vi "YKMW100 Clear Output Buffer.vi"(0 "VISA session":refnum<visa-resource-name>="MW100", 11 "error in (no error)":errorcluster) -> (4 "dup VISA session":refnum<visa-resource-name>, 15 "error out":errorcluster)   [LabVIEW 2023]
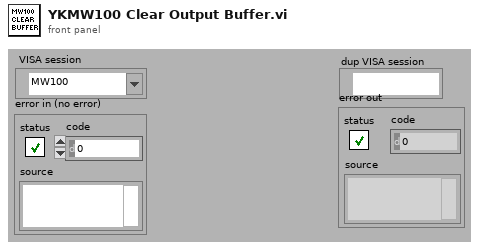
[diagram p1: front panel]
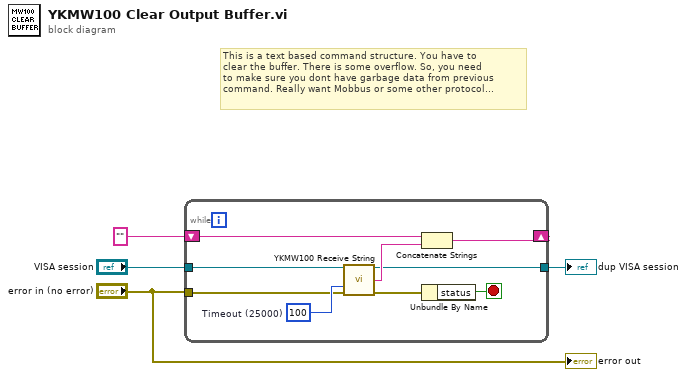
[diagram p0: block diagram]
diagram:
  # "This is a text based command structure. You have to \nclear the buffer. There is some overflow. So, you need\nto make sure you dont have garbage data from previous \ncommand. Really want Mobbus or some other protocol..."
  n1 = while {
    tunnel: "error in (no error)" -> [w11]
    shift-right: [w8] -> _
    shift-left: "" -> [w9]
    tunnel: [w7] -> w3
    tunnel: "VISA session" -> [w5]
    stop <- w13 stop-if-true
    w12 = u32 100  # Timeout (25000)
    n2 = call "YKMW100 Receive String.vi"("VISA session"=w5, "Timeout (25000)"=w12, "error in (no error)"=w11) -> ("dup VISA session"=w7:refnum<visa-resource-name>, "Read Buffer"=w10:string, "error out"=w6:errorcluster)  [unwired: 10 in]
    n3 = Concatenate Strings(w9, w10) -> (w8:string)
    n4 = Unbundle By Name(w6) -> ("status"=w13:bool)
  }
  "dup VISA session" <- w3
  "error out" <- "error in (no error)"
